vi "Set speed.vi"(8 "error in (no error)":errorcluster, 11 "StageSPIM in":refnum<class "StageSPIM.lvclass">) -> (0 "error out":errorcluster, 3 "StageSPIM out":refnum<class "StageSPIM.lvclass">)   [LabVIEW 2012, in "StageSPIM.lvclass"]
uses:
  StageSPIM.lvclass
  StageSPIM.lvclass/StageSPIM.ctl
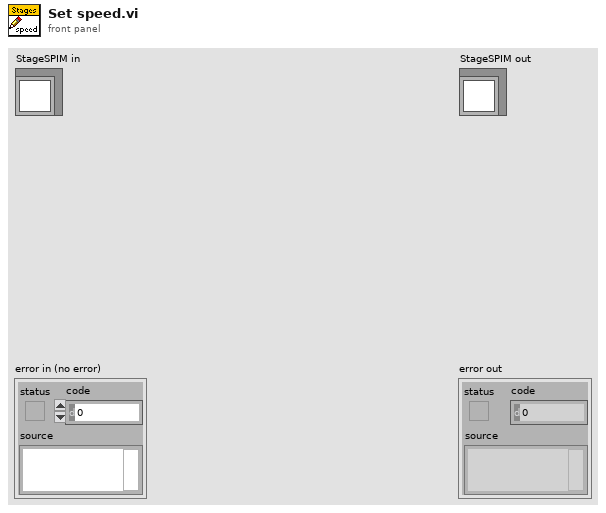
[diagram p1: front panel]
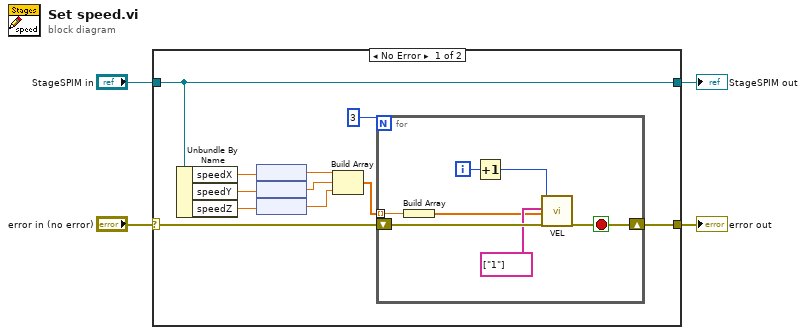
[diagram p0: block diagram]
diagram:
  n1 = case shown="No Error" "error in (no error)" {
    selector: "error in (no error)" -> [w15 w24]
    tunnel: [w14 w24] -> w3
    tunnel: [w12 w23] -> w1
    tunnel: "StageSPIM in" -> [w12 w23]
    frame No Error {
      n2 = Unbundle By Name(w12) -> ("speedX"=w9:dbl[unit], "speedY"=w11:dbl[unit], "speedZ"=w10:dbl[unit])
      n3 = node(w9) -> (w8:dbl)
      n4 = node(w11) -> (w7:dbl)
      n5 = node(w10) -> (w6:dbl)
      n6 = Build Array(w8, w7, w6) -> (w5:dbl[])
      n7 = for {
        N: 3 -> [_]
        shift-right: [w18] -> w14
        shift-left: w15 -> [w22]
        tunnel: w5 -> [w17] mode=indexing
        i -> [w20]
        stop <- w18 stop-if-true
        n8 = Build Array(w17) -> (w16:dbl[])
        n9 = Increment(x=w20) -> (x+1=w19:i32)
        n10 = call "VEL.vi"("System no."=w19, "Axes to set"=string[] ["1"], "Velocity values"=w16, "error in"=w22) -> ("error out"=w18:errorcluster)  [unwired: 14 in, 1 out]
      }
    }
    frame Error {
    }
  }
  "error out" <- w3
  "StageSPIM out" <- w1
